vi "ExpVar AcqExpCondition.vi"(8 "error in (no error)":errorcluster, 11 "ExpVar in":refnum<class "ExpVar.lvclass">) -> (0 "error out":errorcluster, 1 "ExpCondition":cluster{"Label":string, "Value":variant}[](array[cluster]), 3 "ExpVar out":refnum<class "ExpVar.lvclass">)   [LabVIEW 2018, in "ExpVar.lvclass"]
uses:
  ExpVar.lvclass
  ExpVar.lvclass/ExpVar.ctl
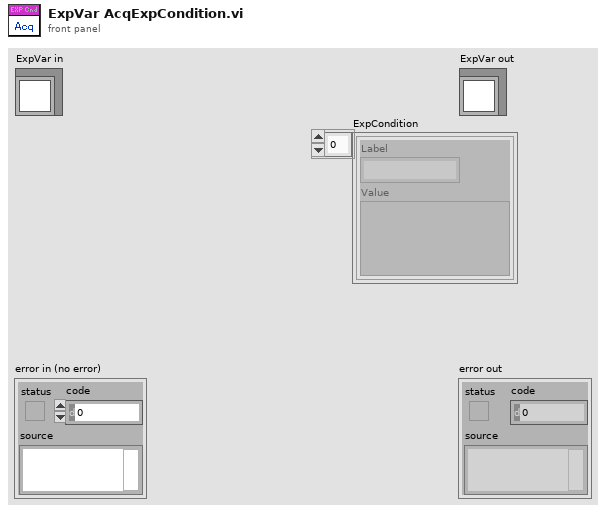
[diagram p1: front panel]
types:
  T1 = cluster{cluster{"Label":string, "Value":variant}[]}[]
  T2 = cluster{cluster{"Label":string, "Value":variant}[]}
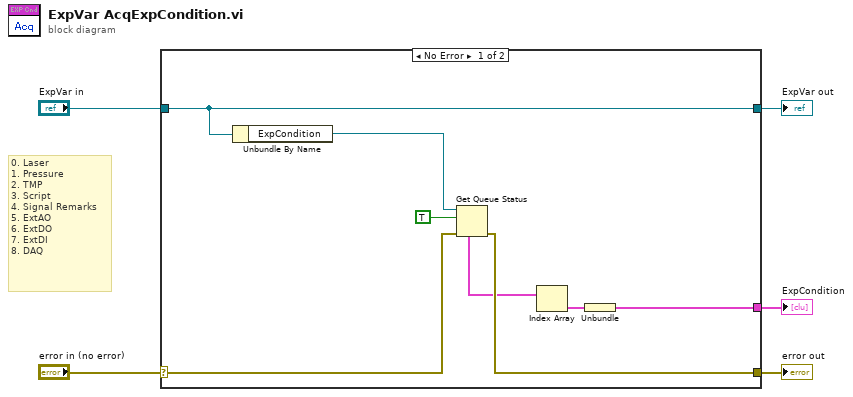
[diagram p0: block diagram]
diagram:
  # "0. Laser\n1. Pressure\n2. TMP\n3. Script\n4. Signal Remarks\n5. ExtAO\n6. ExtDO\n7. ExtDI\n8. DAQ"
  n1 = case shown="No Error" "error in (no error)" {
    selector: "error in (no error)" -> [w11 w15]
    tunnel: [w10 w15] -> w4
    tunnel: [w13 w14] -> w2
    tunnel: "ExpVar in" -> [w13 w14]
    tunnel: [w6 _] -> w1
    frame No Error {
      n2 = Unbundle By Name(w13) -> ("ExpCondition"=w12:refnum<queue>)
      n3 = Get Queue Status(queue=w12, return elements? (F)=TRUE, error in (no error)=w11) -> (error out=w10:errorcluster, elements=w8:T1)  [unwired: 6 out]
      n4 = Index Array(array=w8) -> (element=w7:T2)  [unwired: 1 in]
      n5 = Unbundle(w7) -> (w6:cluster{"Label":string, "Value":variant}[])
    }
    frame Error {
    }
  }
  "error out" <- w4
  "ExpVar out" <- w2
  "ExpCondition" <- w1
